vi "Read Settings.vi"(8 "Error In":errorcluster) -> (0 "Error Out":errorcluster, 1 "Display Informative Note?":bool, 2 "Process Bold Characters?":bool, 3 "Settings Filepath":path)   [LabVIEW 2022 SP3]
doc: "This VI reads the value of the ProcessBoldCharacters and DisplayInformativeNoteWhenToolTakesLongToExecute settings from the \"<B>Free Label to VI Description.ini</B>\" file."
uses:
  <vilib>/Utility/config.llb/Read Key (Boolean).vi
  <vilib>/Utility/config.llb/NI_LVConfig.lvlib
panel:
  out "Any errors occurred inside the VI?":errorcluster
  # "Development\nControls or indicators that are useful for development or testing, but which are not outputs of the VI."
  # "Input\nInputs to the VI"
  # "Output\nOutputs of the VI"
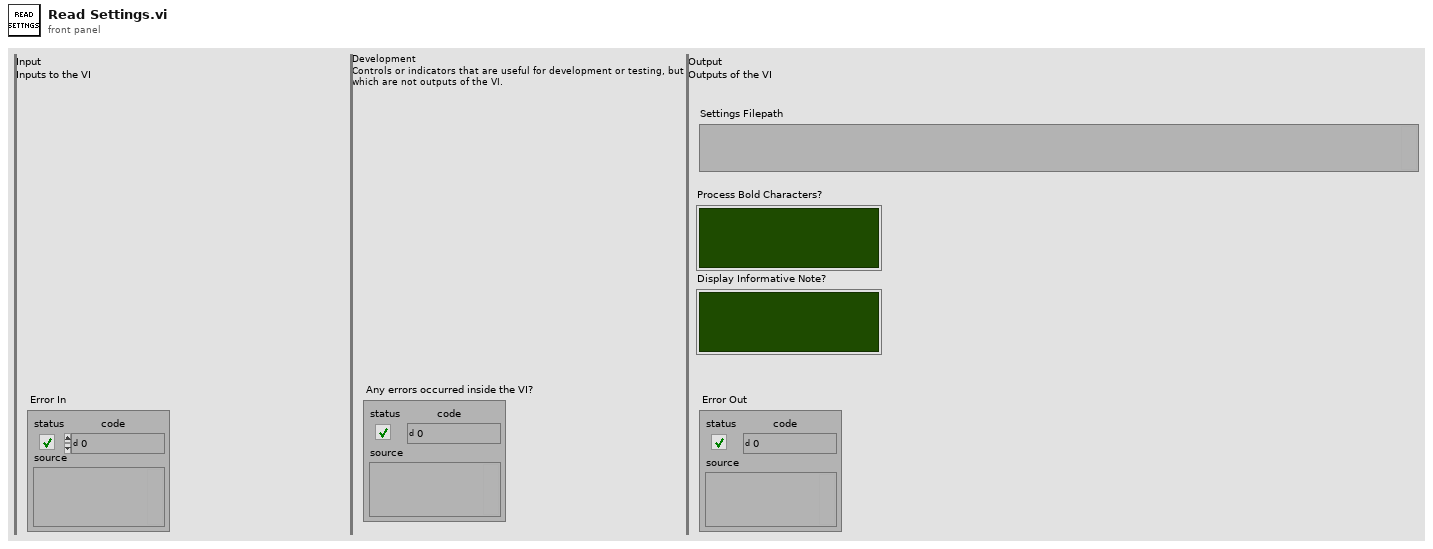
[diagram p1: front panel]
types:
  T1 = typedef "NI_LVConfig.lvlib/Config Data RefNum.ctl" = refnum<k1>
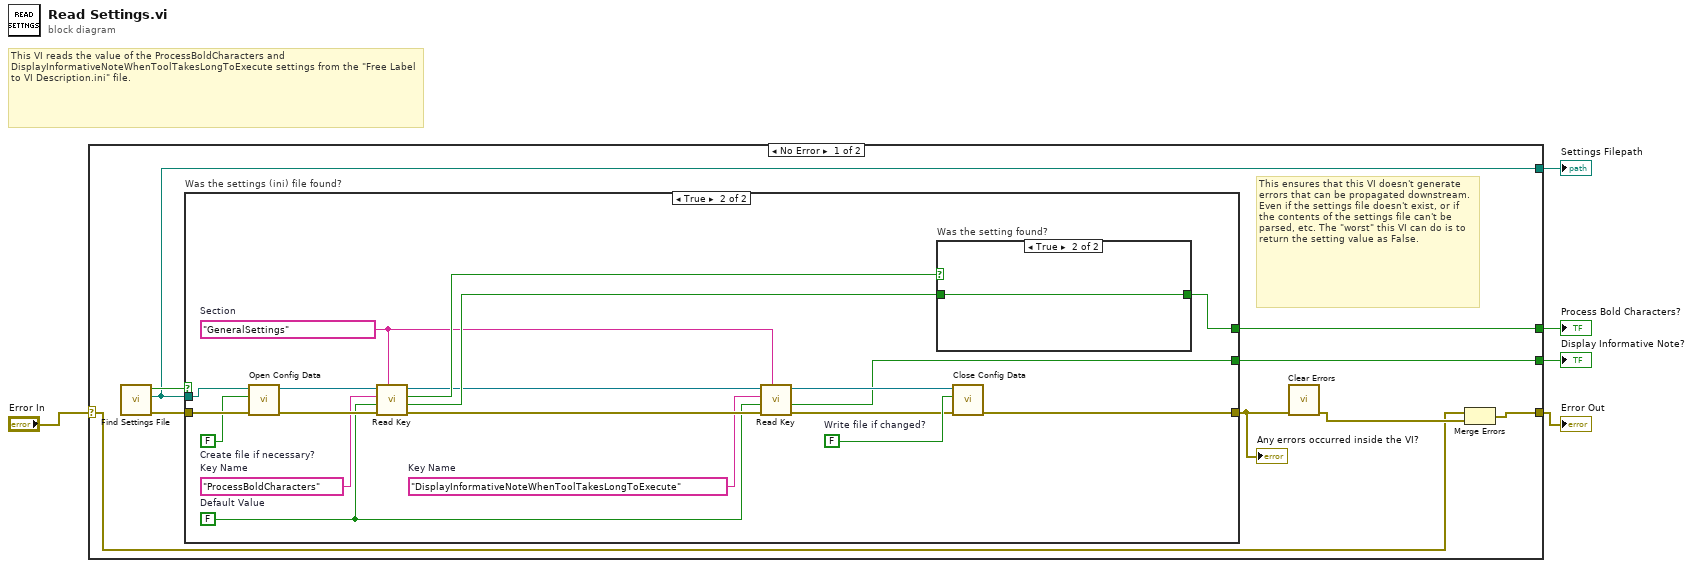
[diagram p0: block diagram]
diagram:
  # "This VI reads the value of the ProcessBoldCharacters and DisplayInformativeNoteWhenToolTakesLongToExecute settings from the \"Free Label to VI Description.ini\" file."
  n1 = case shown="No Error" "Error In" {
    selector: "Error In" -> [w8 w36]
    tunnel: [w10 w36] -> w4
    tunnel: [w11 _] -> w3
    tunnel: [w7 _] -> w2
    tunnel: [w6 _] -> w1
    frame No Error {
      # "This ensures that this VI doesn't generate errors that can be propagated downstream. Even if the settings file doesn't exist, or if the contents of the settings file can't be parsed, etc. The \"worst\" this VI can do is to return the setting value as False."
      n2 = call "Find Settings File.vi"() -> ("Error Out"=w14:errorcluster, "Settings Filepath"=w7:path, "Was settings file found?"=w12:bool)  [unwired: 9 in]
      n3 = case "Was the settings (ini) file found?" shown="True" w12 {
        tunnel: w14 -> [w15 w34]
        tunnel: [w15 w29] -> w13
        tunnel: w7 -> [_ w33]
        tunnel: [_ w24] -> w11
        tunnel: [_ w16] -> w6
        frame False {
          # "If the settings file (ini file)is not found behave as if the settings are all set to False."
        }
        frame True {
          w17 = FALSE  # Default Value
          w18 = "DisplayInformativeNoteWhenToolTakesLongToExecute"  # Key Name
          w27 = "ProcessBoldCharacters"  # Key Name
          w19 = "GeneralSettings"  # Section
          w28 = FALSE  # Write file if changed?
          w32 = FALSE  # Create file if necessary?
          n4 = call <vilib>:"Open Config Data.vi"("error in (no error)"=w34, "create file if necessary (T)"=w32, "configuration file path"=w33) -> ("error out"=w31:errorcluster, "refnum"=w30:T1)  [unwired: 6 in, 1 out]
          n5 = call-poly <vilib>:"Read Key.vi"("section"=w19, "error in (no error)"=w31, "default value"=w17, "key"=w27, "refnum"=w30) -> ("error out"=w23:errorcluster, "value"=w25:bool, "found?"=w26:bool, "refnum out"=w21:T1)  [unwired: 3 in]
          n6 = call-poly <vilib>:"Read Key.vi"("section"=w19, "error in (no error)"=w23, "default value"=w17, "key"=w18, "refnum"=w21) -> ("error out"=w22:errorcluster, "value"=w16:bool, "refnum out"=w20:T1)  [unwired: 3 in, 1 out]
          n7 = case "Was the setting found?" shown="True" w26 {
            tunnel: w25 -> [_ w35]
            tunnel: [_ w35] -> w24
            frame False {
              # "The setting wasn't found. Behave as if the setting is set to False."
            }
            frame True {
            }
          }
          n8 = call <vilib>:"Close Config Data.vi"("error in (no error)"=w22, "write file if changed (T)"=w28, "refnum"=w20) -> ("error out"=w29:errorcluster)  [unwired: 7 in, 1 out]
        }
      }
      "Any errors occurred inside the VI?" <- w13
      n9 = call <vilib>:"Clear Errors.vi"("error in (no error)"=w13) -> ("error out"=w9:errorcluster)  [unwired: 5 in, 1 out]
      n10 = Merge Errors(w8, w9) -> (w10:errorcluster)
    }
    frame Error {
    }
  }
  "Error Out" <- w4
  "Process Bold Characters?" <- w3
  "Settings Filepath" <- w2
  "Display Informative Note?" <- w1
